vi "GetSVNRevision.vi"(11 "File Path Control":path caption="File Path Control (leave blank to use Constants_Global value of EnFlo SW Folder)") -> (0 "This Folder's Last Changed Date":string, 1 "This Folder's Last Revision":string, 2 "LocalModifications":string, 3 "OverallRevision":string, 4 "standard error":string, 5 "standard output":string)   [LabVIEW 2016]
doc: "This VI uses the system's installed svn (subversion) software to return the revision number of the selected folder. Leaving the selected folder blank will use the global value of \"EnFlo SW Folder\".\nThe \"Overall Revision\" is the highest revision number in the entire hierarchy, recursing upwards as well as downwards- in other words, the revision which was checked out. The \"This Folder\" data is specific to the last changes to the selected folder."
uses:
  Globals/Constants_global.vi
panel:
  out "This Folder Last Committed By":string
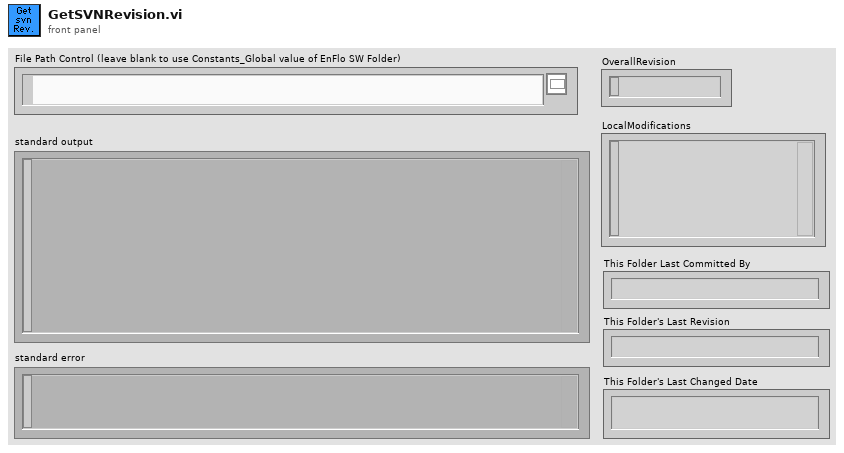
[diagram p1: front panel]
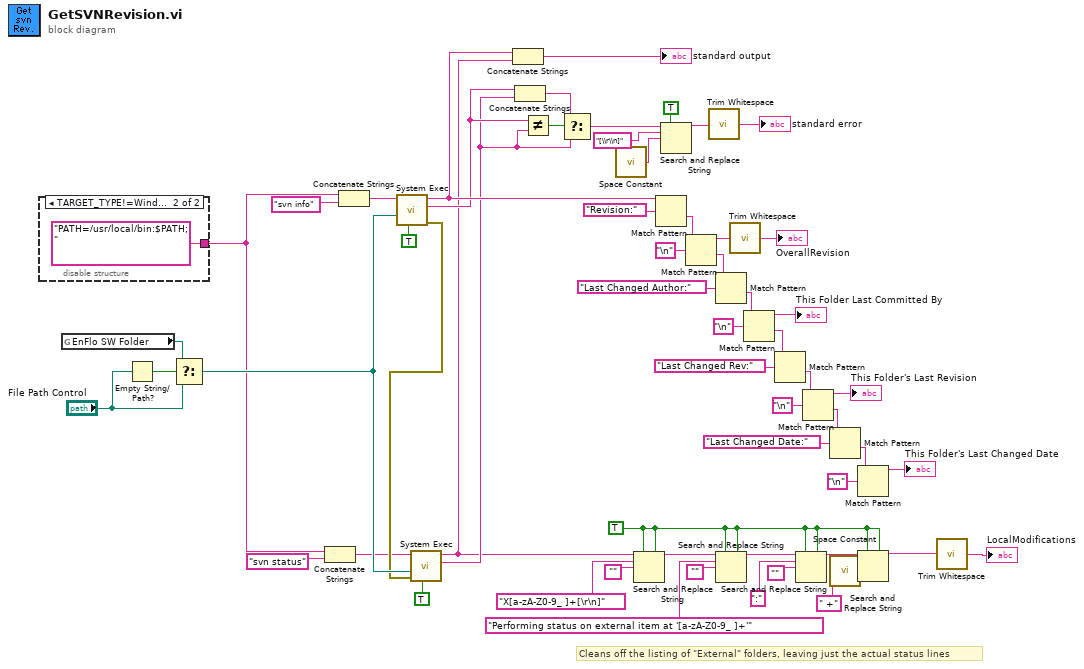
[diagram p0: block diagram]
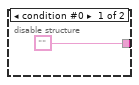
[diagram p2: hidden frame]
diagram:
  w16 = TRUE ("replace all? (F)")
  # "Cleans off the listing of \"External\" folders, leaving just the actual status lines"
  n1 = disable-structure shown="TARGET_TYPE!=Windows" {
    disable-tunnel: ["" ("command line") "PATH=/usr/local/bin:$PATH; " ("command line")] -> w4
    frame condition #0 {
    }
    frame condition #1 (active) {
    }
  }
  n2 = global read "Constants_global.vi" "EnFlo SW Folder"() -> (w57:path)
  n3 = Empty String/Path?(string/path="File Path Control") -> (empty?=w59:bool)
  n4 = Select(t=w57, s=w59, f="File Path Control") -> (s? t:f=w36:path)
  n5 = Concatenate Strings(w4, "svn status" ("command line")) -> (w6:string)
  n6 = Concatenate Strings(w4, "svn info" ("command line")) -> (w8:string)
  n7 = call <vilib>:"System Exec.vi"("run minimized? (F)"=TRUE, "working directory"=w36, "command line"=w8) -> ("error out"=w34:errorcluster, "standard error"=w31:string, "standard output"=w56:string)  [unwired: 5 in, 1 out]
  n8 = call <vilib>:"System Exec.vi"("run minimized? (F)"=TRUE, "error in (no error)"=w34, "working directory"=w36, "command line"=w6) -> ("standard error"=w28:string, "standard output"=w1:string)  [unwired: 4 in, 2 out]
  n9 = Concatenate Strings(w56, w1) -> (→"standard output":string)
  n10 = Concatenate Strings(w31, w28) -> (w29:string)
  n11 = Not Equal?(x=w31, y=w28) -> (x != y?=w30:bool)
  n12 = Select(t=w29, s=w30, f=w28) -> (s? t:f=w10:string)
  n13 = call <vilib>:"Space Constant.vi"() -> ("String"=w12:string)
  n14 = Search and Replace String(replace all?=w16, multiline?=w16, input string=w1, search string="X[a-zA-Z0-9_ ]+[\r\n]", replace string="") -> (result string=w23:string)  [unwired: 3 in, 3 out]
  n15 = Match Pattern(string=w56, regular expression="Revision:") -> (after substring=w54:string)  [unwired: 1 in, 3 out]
  n16 = Search and Replace String(replace all?=TRUE ("replace all? (F)"), input string=w10, search string="[\\r\\n]", replace string=w12) -> (result string=w9:string)  [unwired: 4 in, 3 out]
  n17 = Match Pattern(string=w54, regular expression="\n") -> (before substring=w52:string, after substring=w51:string)  [unwired: 1 in, 2 out]
  n18 = call <vilib>:"Trim Whitespace.vi"("string"=w9) -> ("trimmed string"=→"standard error":string)  [unwired: 1 in]
  n19 = Match Pattern(string=w51, regular expression="Last Changed Author:") -> (after substring=w48:string)  [unwired: 1 in, 3 out]
  n20 = Search and Replace String(replace all?=w16, multiline?=w16, input string=w23, search string="Performing status on external item at '[a-zA-Z0-9_ ]+'", replace string="") -> (result string=w21:string)  [unwired: 3 in, 3 out]
  n21 = call <vilib>:"Trim Whitespace.vi"("string"=w52) -> ("trimmed string"=→"OverallRevision":string)  [unwired: 1 in]
  n22 = Match Pattern(string=w48, regular expression="\n") -> (before substring=→"This Folder Last Committed By":string, after substring=w44:string)  [unwired: 1 in, 2 out]
  n23 = Match Pattern(string=w44, regular expression="Last Changed Rev:") -> (after substring=w46:string)  [unwired: 1 in, 3 out]
  n24 = Search and Replace String(replace all?=w16, multiline?=w16, input string=w21, search string=":", replace string="") -> (result string=w18:string)  [unwired: 3 in, 3 out]
  n25 = Match Pattern(string=w46, regular expression="\n") -> (before substring=→"This Folder's Last Revision":string, after substring=w39:string)  [unwired: 1 in, 2 out]
  n26 = Match Pattern(string=w39, regular expression="Last Changed Date:") -> (after substring=w40:string)  [unwired: 1 in, 3 out]
  n27 = call <vilib>:"Space Constant.vi"() -> ("String"=w14:string)
  n28 = Match Pattern(string=w40, regular expression="\n") -> (before substring=→"This Folder's Last Changed Date":string)  [unwired: 1 in, 3 out]
  n29 = Search and Replace String(replace all?=w16, multiline?=w16, input string=w18, search string=" +", replace string=w14) -> (result string=w17:string)  [unwired: 3 in, 3 out]
  n30 = call <vilib>:"Trim Whitespace.vi"("string"=w17) -> ("trimmed string"=→"LocalModifications":string)  [unwired: 1 in]
